vi "Intersect ranges.vi"(1 "range 2":cluster{"min":i16, "max":i16}, 2 "range 1":cluster{"min":i16, "max":i16}) -> (0 "intersection range":cluster{"min":i16, "max":i16})   [LabVIEW 2011, in "COSYLib.lvlib"]
uses:
  COSYLib.lvlib
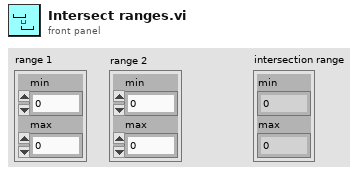
[diagram p1: front panel]
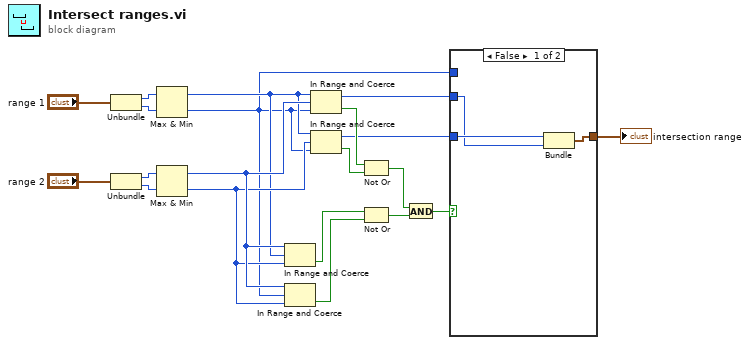
[diagram p0: block diagram]
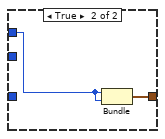
[diagram p2: hidden frame]
diagram:
  n1 = Unbundle("range 1") -> ("min"=w20:i16, "max"=w19:i16)
  n2 = Unbundle("range 2") -> ("min"=w18:i16, "max"=w17:i16)
  n3 = Max & Min(x=w20, y=w19) -> (max(x,y)=w5:i16, min(x,y)=w1:i16)
  n4 = Max & Min(x=w18, y=w17) -> (max(x,y)=w14:i16, min(x,y)=w13:i16)
  n5 = In Range and Coerce(upper limit=w14, x=w5, lower limit=w13) -> (In Range?=w12:bool)  [unwired: 1 out]
  n6 = In Range and Coerce(upper limit=w14, x=w1, lower limit=w13) -> (In Range?=w11:bool)  [unwired: 1 out]
  n7 = In Range and Coerce(upper limit=w5, x=w14, lower limit=w1) -> (coerced(x)=w4:i16, In Range?=w9:bool)
  n8 = In Range and Coerce(upper limit=w5, x=w13, lower limit=w1) -> (coerced(x)=w3:i16, In Range?=w10:bool)
  n9 = Not Or(1:w10, 2:w9) -> (0:w8:bool)
  n10 = Not Or(1:w11, 2:w12) -> (0:w7:bool)
  n11 = And(x=w8, y=w7) -> (x .and. y?=w6:bool)
  n12 = case shown="False" w6 {
    tunnel: w1 -> [_ w25]
    tunnel: w4 -> [w21 _]
    tunnel: w3 -> [w22 _]
    tunnel: [w23 w24] -> w2
    frame False {
      n13 = Bundle(w22, w21) -> (w23:cluster{i16, i16})  [unwired: 1 in]
    }
    frame True {
      n14 = Bundle(w25, w25) -> (w24:cluster{i16, i16})  [unwired: 1 in]
    }
  }
  "intersection range" <- w2
